vi "Conversion Temperature.vi"(8 "error in (no error)":errorcluster, 10 "Input":dbl, 11 "Top Level in":refnum<class "Top Level.lvclass">) -> (0 "error out":errorcluster, 2 "Output":dbl, 3 "Top Level out":refnum<class "Top Level.lvclass">)   [LabVIEW 2021, in "Top Level.lvlib" / "Top Level.lvclass"]
uses:
  Top Level.lvclass
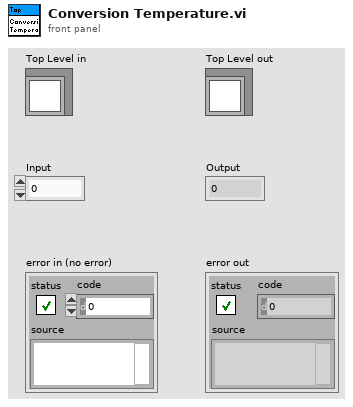
[diagram p1: front panel]
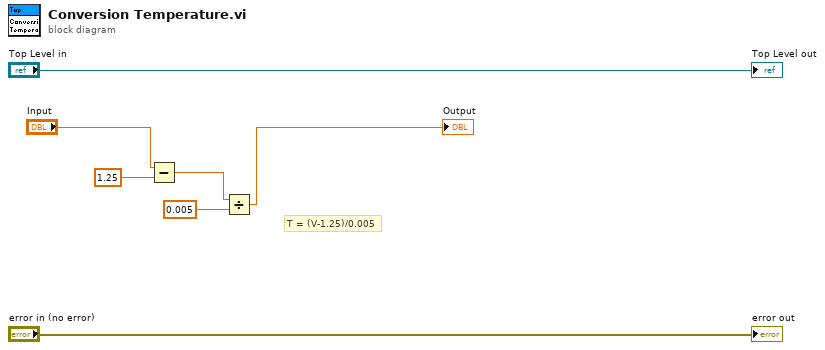
[diagram p0: block diagram]
diagram:
  # "T = (V-1.25)/0.005"
  n1 = Subtract(x="Input", y=1.25) -> (x-y=w4:dbl)
  n2 = Divide(x=w4, y=0.005) -> (x/y=→"Output":dbl)
  "error out" <- "error in (no error)"
  "Top Level out" <- "Top Level in"
